vi "get Available Data.vi"(8 "error in (no error)":errorcluster, 9 "data_number":u32, 10 "Board":u16, 11 "identifier":string) -> (0 "error out":errorcluster, 1 "data_number out":u32, 3 "function return":bool)   [LabVIEW 2015, in "XGL_DPP.lvlib"]
doc: "EXTERN DECLSPEC bool CALL_CONV getAvailableData(const char * identifier,\n uint16_t Board,\n uint32_t * data_number\n);"
uses:
  XGL_DPP.lvlib
  XGL_DPP.dll
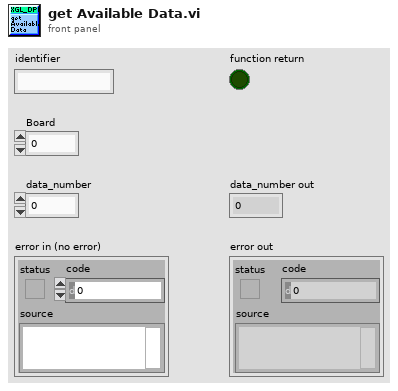
[diagram p1: front panel]
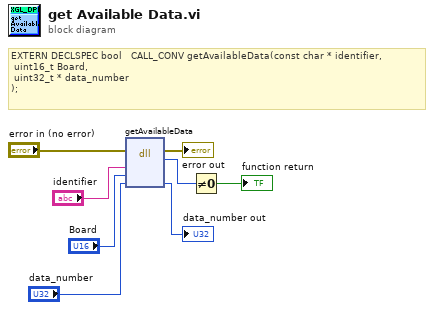
[diagram p0: block diagram]
diagram:
  # "EXTERN DECLSPEC bool   CALL_CONV getAvailableData(const char * identifier,\n\tuint16_t Board,\n\tuint32_t * data_number\n);"
  n1 = dll-call lib="D:/Users/XRF/Desktop/Scanning Software_Demokritos_2015_v7/libs/Vis_2/XGL_DPP.*" fn="getAvailableData"(error in="error in (no error)", "identifier"="identifier", "Board"="Board", "data_number"="data_number") -> (error out=→"error out":errorcluster, w7:u8, "data_number"=→"data_number out":u32)  [unwired: 4 in, 1 out]
  n2 = Not Equal To 0?(x=w7) -> (x != 0?=→"function return":bool)
